vi "IMAQdx Wait for PnP Event.vi"(7 "Timeout (ms)":i32=5000, 8 "error in":errorcluster, 10 "Event":u32(ring) items=["Camera Attached", "Camera Detached", "Bus Reset"], 11 "Session In":T1) -> (0 "error out":errorcluster, 3 "Session Out":T1)   [LabVIEW 2020, in "NI_Vision_Acquisition_Software.lvlib"]
doc: "Synchronous wait for a Plug-and-Play event."
uses:
  NI_Vision_Acquisition_Software.lvlib
  IMAQdx.ctl
  niimaqdx.dll
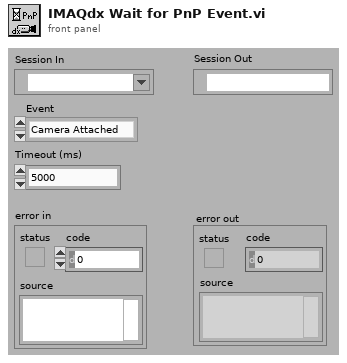
[diagram p1: front panel]
types:
  T1 = typedef "IMAQdx.ctl" = refnum<k21>
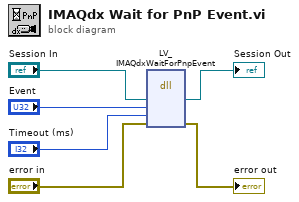
[diagram p0: block diagram]
diagram:
  n1 = dll-call lib="niimaqdx.dll" fn="LV_IMAQdxWaitForPnpEvent"("refnum"="Session In", "event"="Event", "timeoutMs"="Timeout (ms)", "error"="error in") -> ("refnum"=→"Session Out":T1, "error"=→"error out":errorcluster)  [unwired: 6 in, 2 out]
